vi "Agilent34401AInit.vi"(8 "error in (no error)":errorcluster) -> (0 "error out":errorcluster)   [LabVIEW 2014]
uses:
  FGV.ctl
  <instrlib>/Agilent 34401/Agilent 34401.lvlib
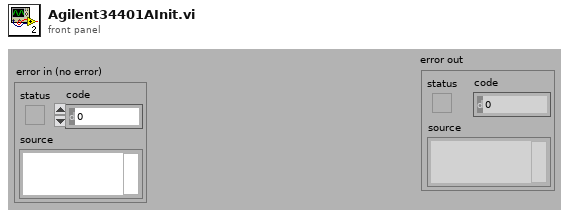
[diagram p1: front panel]
types:
  T1 = typedef "FGV.ctl" = enum16{"Write", "Read", "Init"}
  T2 = typedef "Agilent34401AData.ctl" = cluster{"Adress":refnum<visa-resource-name>}
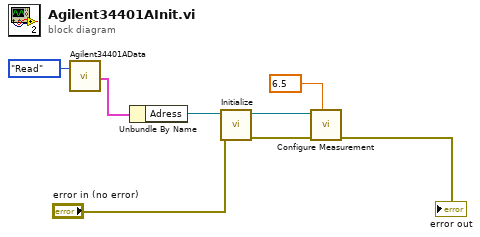
[diagram p0: block diagram]
diagram:
  w1 = 6.5 items=["4.5"=4.5, "5.5"=5.5, "6.5"=6.5] ("Manual Resolution (5.5 Digits)")
  n1 = call "Agilent34401AData.vi"("Enum"=FGV."Read") -> ("Cluster 2"=w7:T2)  [unwired: 17 in, 1 out]
  n2 = Unbundle By Name(w7) -> ("Adress"=w6:refnum<visa-resource-name>)
  n3 = call <instrlib>:"Initialize.vi"("error in (no error)"="error in (no error)", "VISA resource name"=w6) -> ("error out"=w3:errorcluster, "VISA resource name out"=w4:refnum<visa-resource-name>)  [unwired: 8 in]
  n4 = call <instrlib>:"Configure Measurement.vi"("Manual Resolution (5.5 Digits)"=w1, "error in (no error)"=w3, "VISA resource name"=w4) -> ("error out"=→"error out":errorcluster)  [unwired: 7 in, 1 out]
